vi "Demo Plugin.vi"() -> ()   [LabVIEW 2014]
uses:
  DriverMaster/build/DriverMaster.lvlibp/DriverMasterClass/DriverMaster.lvclass
  <vilib>/Utility/LVLibp/NI_PackedLibraryUtility.lvlib
panel:
  in  "REFRESH":bool
  in  "Iniciar Driver":bool
  in  "Drivers Disponibles":string(combo)
  in  "Directorio de Drivers":path
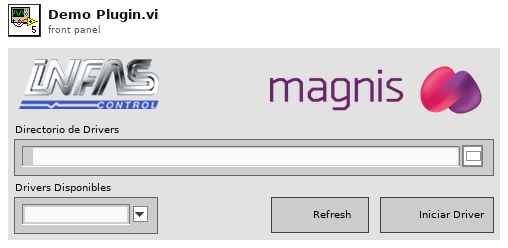
[diagram p1: front panel]
types:
  T1 = enum32{"invalid app kind", "Development System", "Run Time System", "Student Edition", "Embedded LabVIEW", "Evaluation", "Custom"}
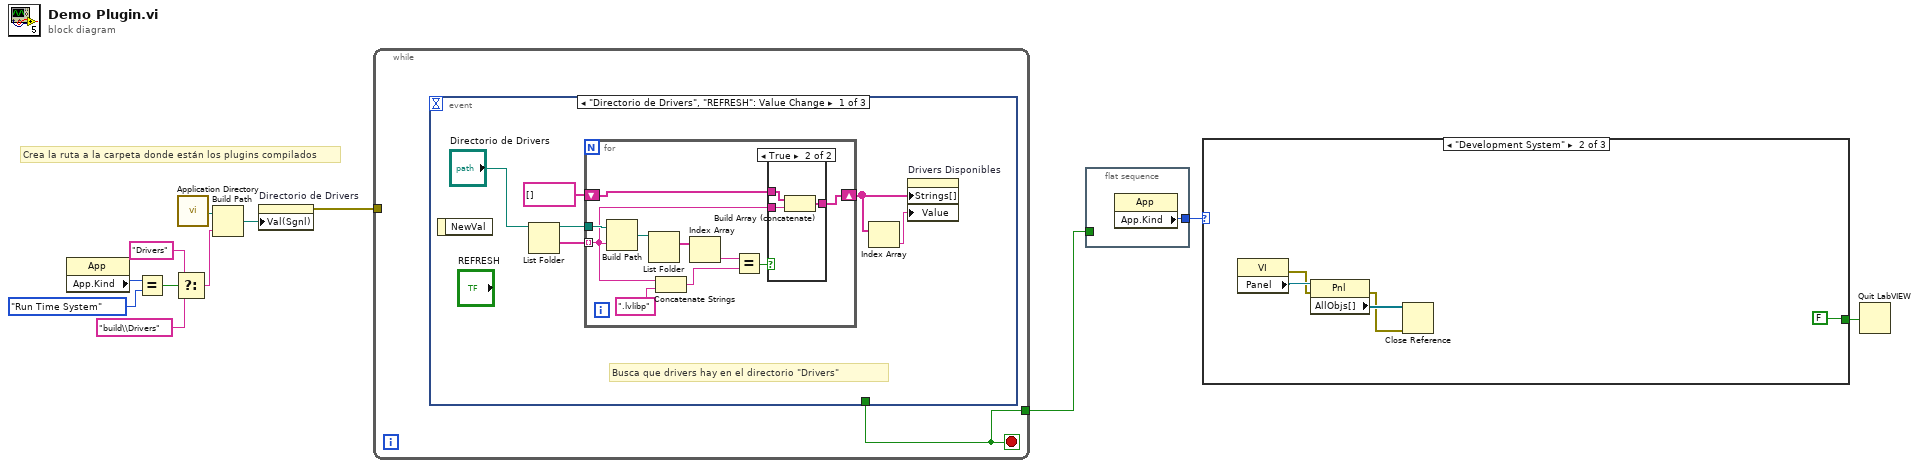
[diagram p0: block diagram]
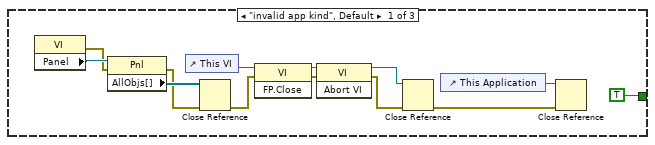
[diagram p2: hidden frame]
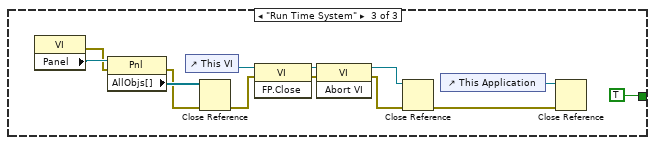
[diagram p3: hidden frame]
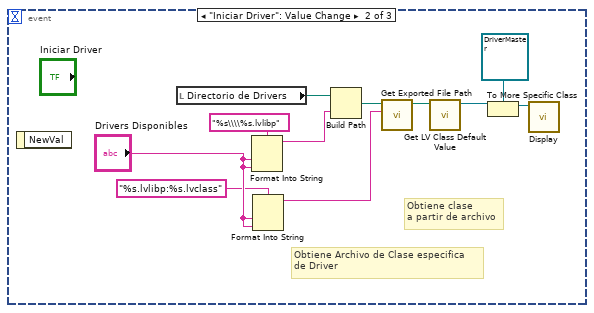
[diagram p5: hidden frame]
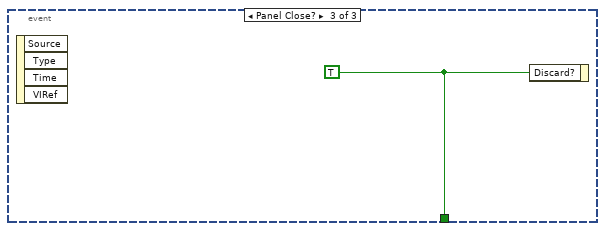
[diagram p6: hidden frame]
diagram:
  # "Crea la ruta a la carpeta donde están los plugins compilados"
  n1 = property class="App"() -> ("App.Kind"=w11:T1)  [unwired: 2 in, 2 out]
  n2 = Equal?(x=w11, y=T1."Run Time System") -> (x = y?=w9:bool)
  n3 = Select(t="Drivers" ("name or relative path"), s=w9, f="build\\Drivers" ("name or relative path")) -> (s? t:f=w6:string)
  n4 = call <vilib>:"Application Directory.vi"() -> ("Application Directory"=w12:path)
  n5 = Build Path(base path=w12, name or relative path=w6) -> (appended path=w5:path)
  n6 = property on="Directorio de Drivers" class="Path"("Val(Sgnl)"=w5) -> (error out=w1:errorcluster)  [unwired: 2 in, 1 out]
  n7 = while {
    tunnel: [w13] -> w2
    tunnel: w1 -> [_]
    stop <- w13 stop-if-true
    n8 = event shown="[0] \"Directorio de Drivers\", \"REFRESH\": Value Change" {
      selector: _ -> [_ _ _]
      dyn-events: _ -> [_ _ _]
      timeout: _ -> [_ _ _]
      tunnel: [_ _ w45] -> w13
      event "Directorio de Drivers", "REFRESH": Value Change {
        # "Busca que drivers hay en el directorio \"Drivers\""
        n9 = event-data() -> ()  [unwired: 1 in, 1 out]
        n10 = List Folder(path="Directorio de Drivers") -> (path out=w18:path, folder names=w17:string[])  [unwired: 3 in, 2 out]
        n11 = for {
          tunnel: w17 -> [w22] mode=indexing
          tunnel: w18 -> [w29]
          shift-right: [w20] -> w16
          shift-left: string[] [] -> [w21]
          n12 = Build Path(base path=w29, name or relative path=w22) -> (appended path=w28:path)
          n13 = List Folder(path=w28) -> (filenames=w27:string[])  [unwired: 3 in, 3 out]
          n14 = Concatenate Strings(w22, ".lvlibp" ("string")) -> (w24:string)
          n15 = Index Array(array=w27) -> (element=w26:string)  [unwired: 1 in]
          n16 = Equal?(x=w26, y=w24) -> (x = y?=w23:bool)
          n17 = case shown="True" w23 {
            tunnel: w22 -> [_ w33]
            tunnel: w21 -> [w30 w32]
            tunnel: [w30 w31] -> w20
            frame False {
            }
            frame True {
              n18 = Build Array (concatenate)(w32, w33) -> (w31:string[])
            }
          }
        }
        n19 = Index Array(array=w16) -> (element=w15:string)  [unwired: 1 in]
        n20 = property on="Drivers Disponibles" class="CmbBox"("Strings[]"=w16, "Value"=w15) -> ()  [unwired: 2 in, 2 out]
      }
      event "Iniciar Driver": Value Change {
        # "Obtiene clase\na partir de archivo"
        # "Obtiene Archivo de Clase especifica\nde Driver"
        n21 = event-data() -> ()  [unwired: 1 in, 1 out]
        n22 = local read "Directorio de Drivers"() -> (w34:path)
        n23 = Format Into String(format string="%s\\\\%s.lvlibp", "Drivers Disponibles", "Drivers Disponibles") -> (resulting string=w43:string)  [unwired: 2 in, 1 out]
        n24 = Format Into String(format string="%s.lvlibp:%s.lvclass", "Drivers Disponibles", "Drivers Disponibles") -> (resulting string=w40:string)  [unwired: 2 in, 1 out]
        n25 = Build Path(base path=w34, name or relative path=w43) -> (appended path=w42:path)
        n26 = call <vilib>:"Get Exported File Path.vi"("qualified name"=w40, "packed library path"=w42) -> ("path"=w41:path)  [unwired: 8 in, 1 out]
        n27 = call <vilib>:"Get LV Class Default Value.vi"("class path"=w41) -> ("object"=w39:refnum<class>)  [unwired: 9 in, 1 out]
        n28 = To More Specific Class(target class=refnum<class "DriverMaster.lvclass"> refnum ("DriverMaster.lvlibp:DriverMaster.lvclass"), reference=w39) -> (specific class reference=w36:refnum<class "DriverMaster.lvclass">)  [unwired: 1 in, 1 out]
        n29 = call-dynamic "Display.vi"("DriverMaster in"=w36) -> ()  [unwired: 9 in, 2 out]
      }
      event Panel Close? {
        w45 = TRUE
        n30 = event-data() -> ()  [unwired: 1 in, 4 out]
        n31 = event-data("Discard?"=w45) -> ()  [unwired: 1 in, 1 out]
      }
    }
  }
  n32 = flat-sequence {
    tunnel: [w46] -> w4
    tunnel: w2 -> [_]
    frame #0 {
      n33 = property class="App"() -> ("App.Kind"=w46:T1)  [unwired: 2 in, 2 out]
    }
  }
  n34 = case shown="\"Development System\"" w4 {
    tunnel: [TRUE FALSE TRUE] -> w3
    frame "invalid app kind", Default {
      n35 = property class="VI"() -> (error out=w47:errorcluster, "Panel"=w57:refnum<vi>)  [unwired: 2 in, 1 out]
      n36 = property class="Pnl"(reference=w57, error in=w47) -> (error out=w48:errorcluster, "AllObjs[]"=w56:refnum<vi>[])  [unwired: 1 out]
      n37 = control-ref of="This VI"() -> (w54:refnum<vi>)
      n38 = Close Reference(reference=w56, error in (no error)=w48) -> (error out=w53:errorcluster)
      n39 = invoke class="VI" method="FP.Close"(reference=w54, error in=w53) -> (reference out=w52:refnum<vi>, error out=w51:errorcluster)  [unwired: 1 in, 1 out]
      n40 = invoke class="VI" method="Abort VI"(reference=w52, error in=w51) -> (reference out=w49:refnum<vi>, error out=w50:errorcluster)  [unwired: 1 in, 1 out]
      n41 = Close Reference(reference=w49, error in (no error)=w50) -> (error out=w58:errorcluster)
      n42 = control-ref of="This Application"() -> (w59:refnum<vi>)
      n43 = Close Reference(reference=w59, error in (no error)=w58) -> ()  [unwired: 1 out]
    }
    frame "Development System" {
      n44 = property class="VI"() -> (error out=w60:errorcluster, "Panel"=w64:refnum<vi>)  [unwired: 2 in, 1 out]
      n45 = property class="Pnl"(reference=w64, error in=w60) -> (error out=w61:errorcluster, "AllObjs[]"=w63:refnum<vi>[])  [unwired: 1 out]
      n46 = Close Reference(reference=w63, error in (no error)=w61) -> ()  [unwired: 1 out]
    }
    frame "Run Time System" {
      n47 = property class="VI"() -> (error out=w65:errorcluster, "Panel"=w75:refnum<vi>)  [unwired: 2 in, 1 out]
      n48 = property class="Pnl"(reference=w75, error in=w65) -> (error out=w66:errorcluster, "AllObjs[]"=w74:refnum<vi>[])  [unwired: 1 out]
      n49 = control-ref of="This VI"() -> (w72:refnum<vi>)
      n50 = Close Reference(reference=w74, error in (no error)=w66) -> (error out=w71:errorcluster)
      n51 = invoke class="VI" method="FP.Close"(reference=w72, error in=w71) -> (reference out=w70:refnum<vi>, error out=w69:errorcluster)  [unwired: 1 in, 1 out]
      n52 = invoke class="VI" method="Abort VI"(reference=w70, error in=w69) -> (reference out=w67:refnum<vi>, error out=w68:errorcluster)  [unwired: 1 in, 1 out]
      n53 = Close Reference(reference=w67, error in (no error)=w68) -> (error out=w76:errorcluster)
      n54 = control-ref of="This Application"() -> (w77:refnum<vi>)
      n55 = Close Reference(reference=w77, error in (no error)=w76) -> ()  [unwired: 1 out]
    }
  }
  n56 = Quit LabVIEW(quit? (T)=w3) -> ()
